vi "SystemLink Alarm KPIs - Prototype Code.vi"() -> ()   [LabVIEW 2019]
uses:
  <vilib>/Skyline/Alarm/Library/typedefs/Severity Level.ctl
  <vilib>/Skyline/Alarm/Library/typedefs/Transition.ctl
  <vilib>/Skyline/Alarm/Library/typedefs/Transition Type.ctl
  <vilib>/Skyline/Utilities/Property.ctl
  <vilib>/Skyline/Alarm/Filter Class/NI SystemLink Alarm Filter.lvclass
  <vilib>/Skyline/Alarm/Filter Class/NI SystemLink Alarm Filter.lvclass/NI SystemLink Alarm Filter.ctl
  <vilib>/Skyline/Configuration/Configuration HTTP_class/NI Skyline Configuration HTTP.lvclass/NI Skyline Configuration HTTP.ctl
  <vilib>/Skyline/Alarm/Class/NI SystemLink Alarm.lvclass/NI SystemLink Alarm.ctl
  <vilib>/Analysis/baseanly.llb/Mean (DBL).vi
  <vilib>/Skyline/Alarm/Class/Accessors/Read Acknowledged At.vi
  <vilib>/Skyline/Alarm/Class/Accessors/Read Highest Severity Level.vi
  <vilib>/Skyline/Alarm/Class/Accessors/Read Acknowledged.vi
  <vilib>/Skyline/Alarm/Class/Accessors/Read Active.vi
  <vilib>/Skyline/Alarm/Filter Class/Write Occurred After.vi
  <vilib>/Skyline/Alarm/Filter Class/Read Filter.vi
  <vilib>/Skyline/Configuration/Configuration HTTP_class/Read Configuration.vi
  <vilib>/Skyline/Alarm/Class/Private/Ensure Alarm Information.vi
  <vilib>/Skyline/Alarm/Filter Class/Write Is Active.vi
  <vilib>/Skyline/Alarm/Library/Query Alarms (With Transitions).vi
  <vilib>/Skyline/Alarm/Library/Query Alarms (No Transitions).vi
  <vilib>/Skyline/Alarm/Class/Accessors/Read Transitions.vi
  <vilib>/Skyline/Alarm/Library/Get Alarm Information.vi
  <vilib>/Skyline/Alarm/Filter Class/Write Highest Severity Level Min.vi
  <vilib>/Skyline/Alarm/Filter Class/Write Highest Severity Level Max.vi
  <vilib>/Skyline/Configuration/Configuration HTTP_class/NI Skyline Configuration HTTP.lvclass
  <vilib>/Skyline/Alarm/Class/NI SystemLink Alarm.lvclass
  <vilib>/Skyline/Alarm/Library/NI SystemLink Alarm Library.lvlib
  <vilib>/Analysis/NI_AALBase.lvlib
  <vilib>/Skyline/Utilities/NI Skyline Utilities.lvlib
panel:
  out "Average duration of currently active alarms (HH:MM:SS)":dbl format="%<%H:%M:%S>t"
  out "Average duration of currently active alarms (days)":dbl format="%#.2g"
  out "Average MTTR of inactive alarms (days)":dbl format="%#.2g"
  out "MTTR Array":dbl[](array[numeric]) format="%<%H:%M:%S>t"
  out "Average MTTR of inactive alarms (HH:MM:SS)":dbl format="%<%H:%M:%S>t"
  out "acknowledged?":bool[](array[boolean])
  out "active?":bool[](array[boolean])
  out "acknowledged at":timestamp[](array[timestamp])
  out "Accessors:transitions":T1[][](array[typedef]) {"severity level" items=["Clear (-1)"=-1, "Low (1)"=1, "Moderate (2)"=2, "High (3)"=3, "Critical (4)"=4]}
  out "Array":T3[](array[typedef]) items=["Clear (-1)"=-1, "Low (1)"=1, "Moderate (2)"=2, "High (3)"=3, "Critical (4)"=4]
  out "Start Time":timestamp
  in  "Past n days":dbl
  out "End Time":timestamp
  out "Non-Critical Alarms":i32
  out "Critical Alarms":i32
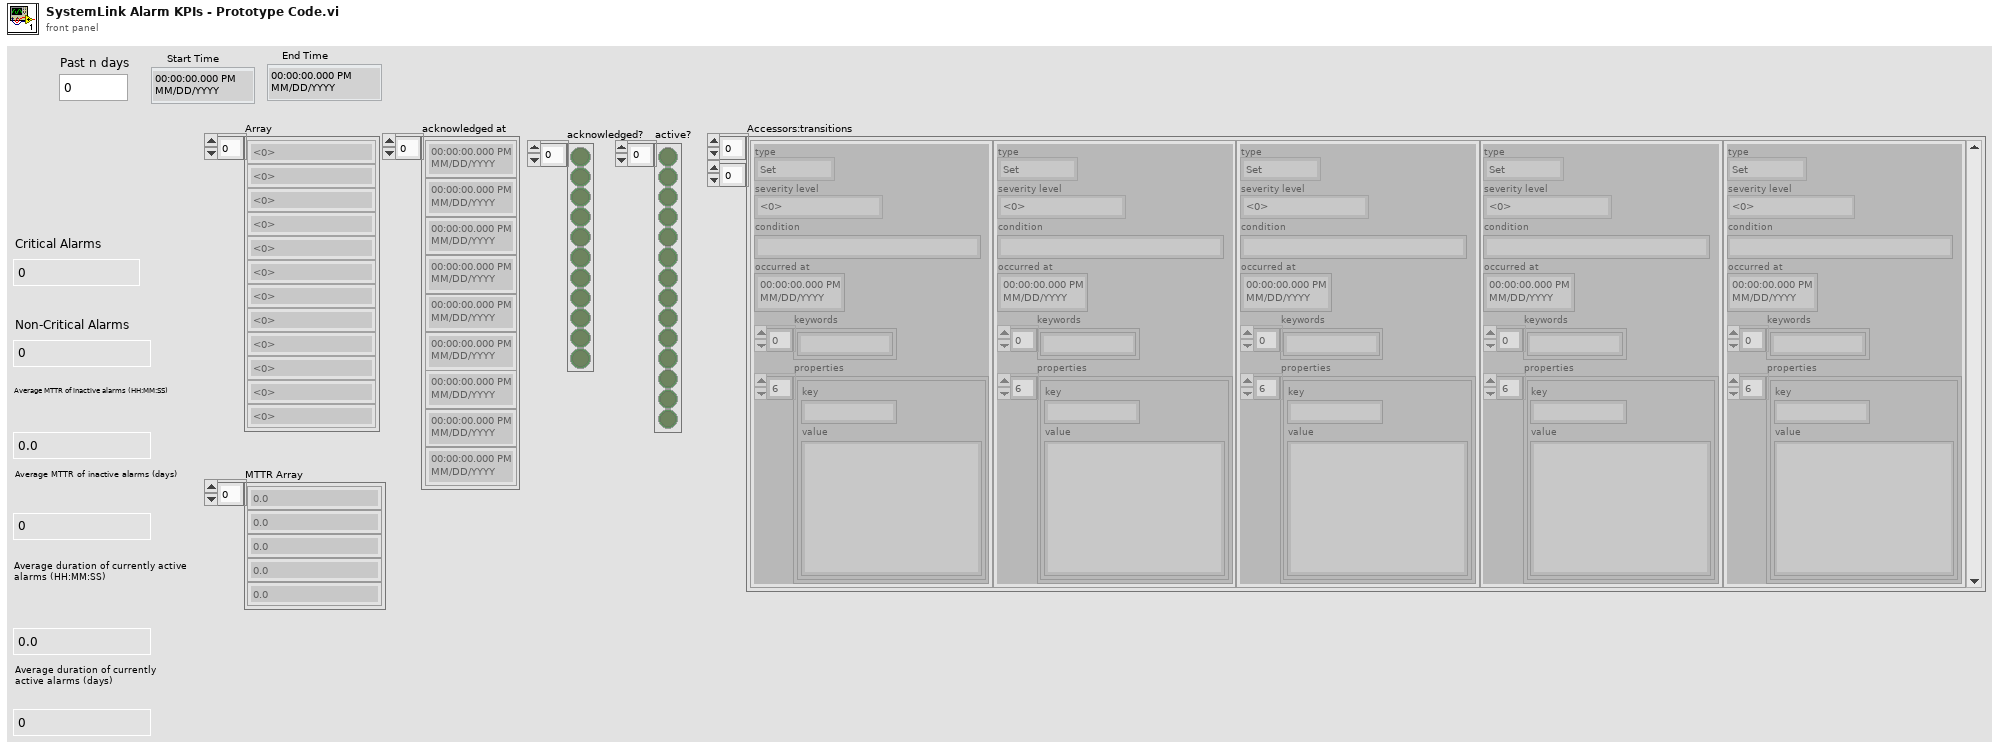
[diagram p1: front panel]
types:
  T1 = typedef "NI SystemLink Alarm Library.lvlib/Transition.ctl" = cluster{"type":T2, "severity level":T3, "condition":string, "occurred at":timestamp, "keywords":string[], "properties":T4[]}
  T2 = typedef "NI SystemLink Alarm Library.lvlib/Transition Type.ctl" = enum16{"Set", "Clear"}
  T3 = typedef "NI SystemLink Alarm Library.lvlib/Severity Level.ctl" = i32
  T4 = typedef "NI Skyline Utilities.lvlib/Property.ctl" = cluster{"key":string, "value":string}
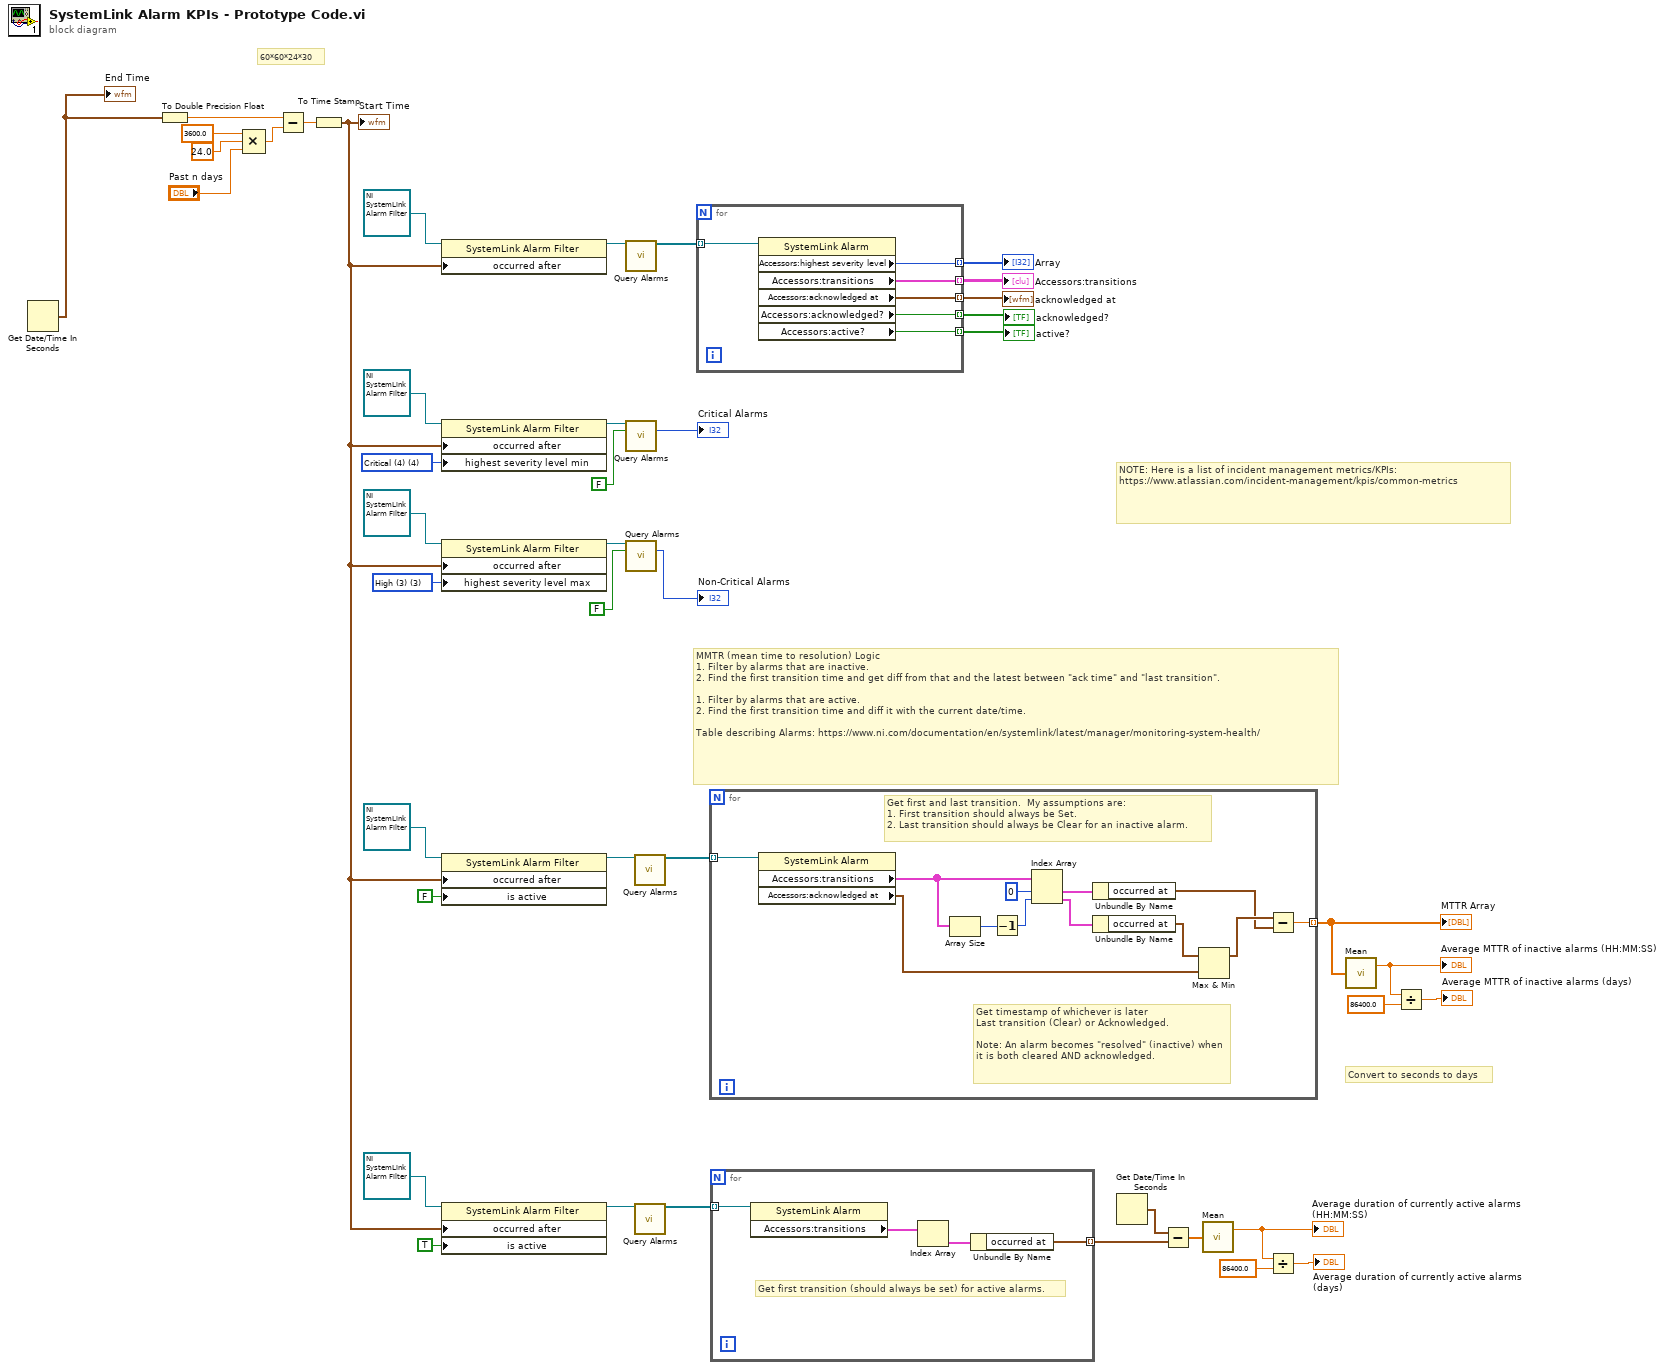
[diagram p0: block diagram]
diagram:
  w29 = T3 4 items=["Clear (-1)"=-1, "Low (1)"=1, "Moderate (2)"=2, "High (3)"=3, "Critical (4)"=4] ("highest severity level max")
  w31 = T3 3 items=["Clear (-1)"=-1, "Low (1)"=1, "Moderate (2)"=2, "High (3)"=3, "Critical (4)"=4] ("highest severity level max")
  # "NOTE: Here is a list of incident management metrics/KPIs:\nhttps://www.atlassian.com/incident-management/kpis/common-metrics"
  # "Convert to seconds to days"
  # "MMTR (mean time to resolution) Logic\n1. Filter by alarms that are inactive.\n2. Find the first transition time and get diff from that and the latest between \"ack time\" and \"last transition\".\n\n1. Filter by alarms that are active.\n2. Find the first transition time and diff it with the current date/time.\n\nTable describing Alarms: https://www.ni.com/documentation/en/systemlink/latest/manager/monitoring-system-health/"
  # "60*60*24*30"
  n1 = Get Date/Time In Seconds() -> (seconds since 1Jan1904=w43:timestamp)
  "End Time" <- w43
  n2 = To Double Precision Float(number=w43) -> (double precision float=w42:dbl)
  n3 = Compound Arithmetic op=MULTIPLY(3600.0 ("value"), 24.0 ("value"), "Past n days") -> (w38:dbl)
  n4 = Subtract(x=w42, y=w38) -> (x-y=w37:dbl)
  n5 = To Time Stamp(1:w37) -> (0:w10:timestamp)
  "Start Time" <- w10
  n6 = property class="SystemLink Alarm Filter"(reference=refnum<class "NI SystemLink Alarm Filter.lvclass"> refnum ("SystemLink Alarm Filter"), "occurred after"=w10) -> (reference out=w35:refnum<class "NI SystemLink Alarm Filter.lvclass">)  [unwired: 1 in, 1 out]
  n7 = property class="SystemLink Alarm Filter"(reference=refnum<class "NI SystemLink Alarm Filter.lvclass"> refnum ("SystemLink Alarm Filter"), "occurred after"=w10, "highest severity level min"=w29) -> (reference out=w27:refnum<class "NI SystemLink Alarm Filter.lvclass">)  [unwired: 1 in, 1 out]
  n8 = property class="SystemLink Alarm Filter"(reference=refnum<class "NI SystemLink Alarm Filter.lvclass"> refnum ("SystemLink Alarm Filter"), "occurred after"=w10, "highest severity level max"=w31) -> (reference out=w34:refnum<class "NI SystemLink Alarm Filter.lvclass">)  [unwired: 1 in, 1 out]
  n9 = property class="SystemLink Alarm Filter"(reference=refnum<class "NI SystemLink Alarm Filter.lvclass"> refnum ("SystemLink Alarm Filter"), "occurred after"=w10, "is active"=FALSE) -> (reference out=w19:refnum<class "NI SystemLink Alarm Filter.lvclass">)  [unwired: 1 in, 1 out]
  n10 = property class="SystemLink Alarm Filter"(reference=refnum<class "NI SystemLink Alarm Filter.lvclass"> refnum ("SystemLink Alarm Filter"), "occurred after"=w10, "is active"=TRUE) -> (reference out=w13:refnum<class "NI SystemLink Alarm Filter.lvclass">)  [unwired: 1 in, 1 out]
  n11 = call <vilib>:"Query Alarms.vi"("filter"=w35) -> ("alarms"=w44:refnum<class "NI SystemLink Alarm.lvclass">[])  [unwired: 12 in, 2 out]
  n12 = call <vilib>:"Query Alarms.vi"("filter"=w27, "retrieve transitions?"=FALSE) -> ("total count"=→"Critical Alarms":i32)  [unwired: 11 in, 2 out]
  n13 = call <vilib>:"Query Alarms.vi"("filter"=w34, "retrieve transitions?"=FALSE) -> ("total count"=→"Non-Critical Alarms":i32)  [unwired: 11 in, 2 out]
  n14 = call <vilib>:"Query Alarms.vi"("filter"=w19) -> ("alarms"=w18:refnum<class "NI SystemLink Alarm.lvclass">[])  [unwired: 12 in, 2 out]
  n15 = call <vilib>:"Query Alarms.vi"("filter"=w13) -> ("alarms"=w9:refnum<class "NI SystemLink Alarm.lvclass">[])  [unwired: 12 in, 2 out]
  n16 = for {
    tunnel: w44 -> [w50] mode=indexing
    tunnel: [w49] -> w32 mode=indexing
    tunnel: [w48] -> w25 mode=indexing
    tunnel: [w47] -> w24 mode=indexing
    tunnel: [w46] -> w23 mode=indexing
    tunnel: [w45] -> w22 mode=indexing
    n17 = property class="SystemLink Alarm"(reference=w50) -> ("Accessors:highest severity level"=w49:T3, "Accessors:transitions"=w48:T1[], "Accessors:acknowledged at"=w47:timestamp, "Accessors:acknowledged?"=w45:bool, "Accessors:active?"=w46:bool)  [unwired: 1 in, 2 out]
  }
  "Array" <- w32
  "Accessors:transitions" <- w25
  "acknowledged at" <- w24
  "active?" <- w23
  "acknowledged?" <- w22
  n18 = for {
    tunnel: w18 -> [w62] mode=indexing
    tunnel: [w51] -> w17 mode=indexing
    # "Get timestamp of whichever is later\nLast transition (Clear) or Acknowledged.\n\nNote: An alarm becomes \"resolved\" (inactive) when it is both cleared AND acknowledged."
    # "Get first and last transition.  My assumptions are:\n1. First transition should always be Set.\n2. Last transition should always be Clear for an inactive alarm."
    n19 = property class="SystemLink Alarm"(reference=w62) -> ("Accessors:transitions"=w60:T1[], "Accessors:acknowledged at"=w54:timestamp)  [unwired: 1 in, 2 out]
    n20 = Array Size(array=w60) -> (size(s)=w59:i32)
    n21 = Decrement(x=w59) -> (x-1=w58:i32)
    n22 = Index Array(array=w60, index #1=0 ("index"), index #2=w58) -> (element #1=w57:T1, element #2=w56:T1)
    n23 = Unbundle By Name(w57) -> ("occurred at"=w52:timestamp)
    n24 = Unbundle By Name(w56) -> ("occurred at"=w55:timestamp)
    n25 = Max & Min(x=w55, y=w54) -> (max(x,y)=w53:timestamp)  [unwired: 1 out]
    n26 = Subtract(x=w53, y=w52) -> (x-y=w51:dbl)
  }
  "MTTR Array" <- w17
  n27 = for {
    tunnel: w9 -> [w66] mode=indexing
    tunnel: [w63] -> w8 mode=indexing
    # "Get first transition (should always be set) for active alarms."
    n28 = property class="SystemLink Alarm"(reference=w66) -> ("Accessors:transitions"=w65:T1[])  [unwired: 1 in, 2 out]
    n29 = Index Array(array=w65) -> (element=w64:T1)  [unwired: 1 in]
    n30 = Unbundle By Name(w64) -> ("occurred at"=w63:timestamp)
  }
  n31 = Get Date/Time In Seconds() -> (seconds since 1Jan1904=w3:timestamp)
  n32 = Subtract(x=w3, y=w8) -> (x-y=w7:dbl[])
  n33 = call-poly <vilib>:"Mean.vi"("X"=w7) -> ("mean"=w4:dbl)  [unwired: 1 out]
  "Average duration of currently active alarms (HH:MM:SS)" <- w4
  n34 = Divide(x=w4, y=86400.0) -> (x/y=→"Average duration of currently active alarms (days)":dbl)
  n35 = call-poly <vilib>:"Mean.vi"("X"=w17) -> ("mean"=w16:dbl)  [unwired: 1 out]
  "Average MTTR of inactive alarms (HH:MM:SS)" <- w16
  n36 = Divide(x=w16, y=86400.0) -> (x/y=→"Average MTTR of inactive alarms (days)":dbl)
